vi "Config Settings FGV.vi"(7 "Command":string, 8 "error in (no error)":errorcluster, 10 "Data in":variant) -> (0 "error out":errorcluster, 2 "Data out":variant)   [LabVIEW 2018, in "Configuration.lvlib"]
uses:
  Configuration.lvlib
  <vilib>/Utility/config.llb/NI_LVConfig.lvlib
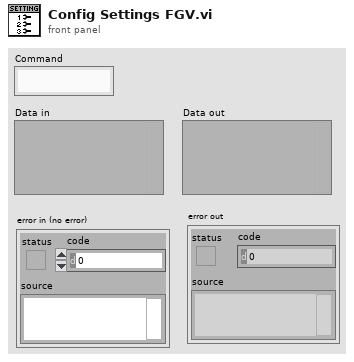
[diagram p1: front panel]
types:
  T1 = typedef "NI_LVConfig.lvlib/Config Data RefNum.ctl" = refnum<k1>
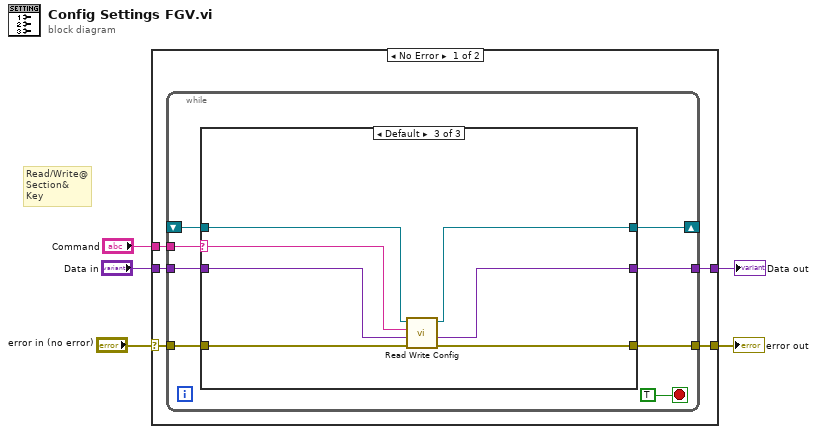
[diagram p0: block diagram]
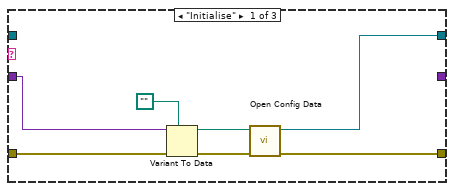
[diagram p2: hidden frame]
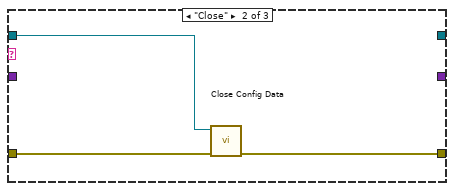
[diagram p3: hidden frame]
diagram:
  # "Read/Write@\nSection&\nKey"
  n1 = case shown="No Error" "error in (no error)" {
    selector: "error in (no error)" -> [w9 w36]
    tunnel: "Command" -> [w10 _]
    tunnel: "Data in" -> [w8 w37]
    tunnel: [w7 w37] -> w2
    tunnel: [w6 w36] -> w1
    frame No Error {
      n2 = while {
        shift-right: [w17] -> _
        shift-left: _ -> [w12]
        tunnel: w10 -> [w16]
        tunnel: w9 -> [w15]
        tunnel: w8 -> [w14]
        tunnel: [w13] -> w7
        tunnel: [w11] -> w6
        stop <- TRUE stop-if-true
        n3 = case shown="Default" w16 {
          selector: w16 -> [_ _ w31]
          tunnel: [w25 _ w30] -> w17
          tunnel: w15 -> [w24 w26 w35]
          tunnel: w14 -> [w22 _ w33]
          tunnel: [_ _ w29] -> w13
          tunnel: w12 -> [_ w28 w32]
          tunnel: [w19 w27 w34] -> w11
          frame "Initialise" {
            n4 = Variant To Data(error in=w24, type=path "" ("configuration file path"), Variant=w22) -> (data=w20:path, error out=w23:errorcluster)
            n5 = call <vilib>:"Open Config Data.vi"("error in (no error)"=w23, "configuration file path"=w20) -> ("error out"=w19:errorcluster, "refnum"=w25:T1)  [unwired: 7 in, 1 out]
          }
          frame "Close" {
            n6 = call <vilib>:"Close Config Data.vi"("error in (no error)"=w26, "refnum"=w28) -> ("error out"=w27:errorcluster)  [unwired: 8 in, 1 out]
          }
          frame Default {
            n7 = call "Read Write Config.vi"("error in (no error)"=w35, "Data in"=w33, "Command"=w31, "config ref in"=w32) -> ("error out"=w34:errorcluster, "Data out"=w29:variant, "config ref out"=w30:T1)  [unwired: 5 in]
          }
        }
      }
    }
    frame Error {
    }
  }
  "Data out" <- w2
  "error out" <- w1
